vi "Day 6.vi"() -> ()   [LabVIEW 2021]
panel:
  out "input":string
  out "input file":path
  out "ouptut 2":u64
  in  "Run [T]/ Example[F]":bool
  out "ouptut 1":u32
  # "Advent of Code 2021 - Day 6 - Lanternfish"
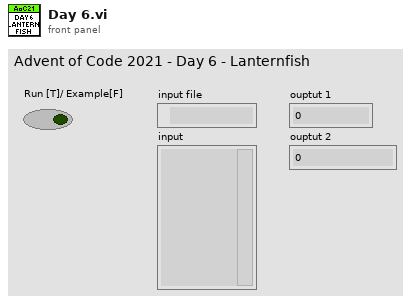
[diagram p1: front panel]
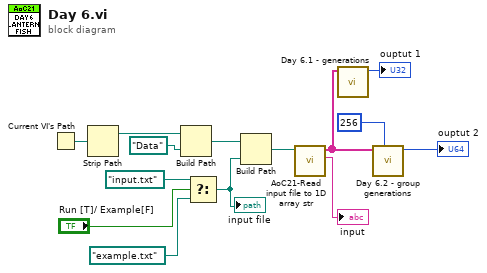
[diagram p0: block diagram]
diagram:
  n1 = Current VI's Path() -> (path=w14:path)
  n2 = Strip Path(path=w14) -> (stripped path=w13:path)  [unwired: 1 out]
  n3 = Build Path(base path=w13, name or relative path=path "Data") -> (appended path=w11:path)
  n4 = Select(t=path "input.txt" ("name or relative path"), s="Run [T]/ Example[F]", f=path "example.txt" ("name or relative path")) -> (s? t:f=w7:path)
  "input file" <- w7
  n5 = Build Path(base path=w11, name or relative path=w7) -> (appended path=w6:path)
  n6 = call "AoC21-Read input file to 1D array str.vi"("input file"=w6) -> ("input text"=→"input":string, "input"=w3:string[])  [unwired: 9 in]
  n7 = call "Day 6.1 - generations.vi"("input"=w3) -> ("output"=→"ouptut 1":u32)  [unwired: 10 in]
  n8 = call "Day 6.2 - group generations.vi"("Generations"=256, "input"=w3) -> ("output"=→"ouptut 2":u64)  [unwired: 9 in]
